vi "Create From Variant (Array).vi"(8 "error in (no error)":errorcluster, 10 "Variant":variant, 11 "JSON Value in":refnum<class "JSON Value.lvclass">) -> (0 "error out":errorcluster, 3 "JSON Value out":refnum<class "JSON Value.lvclass">)   [LabVIEW 2016, in "JSON Value.lvclass"]
doc: "Creates a new JSON instance from the given Variant."
uses:
  JSON Helper/JSON Value.lvclass
  JSON Helper/JSON Value.lvclass/JSON Value.ctl
  JSON Boolean/New JSON Boolean.vi
  JSON String/New JSON String.vi
  JSON Numeric/New JSON Numeric.vi
  <vilib>/Utility/Data Type/NI_Data Type.lvlib
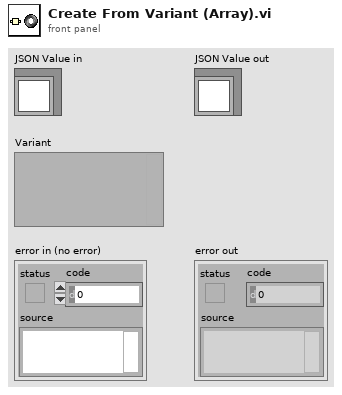
[diagram p1: front panel]
types:
  T1 = typedef "NI_Data Type.lvlib/Data Type.ctl" = enum8{"Invalid Type", "Void", "I8", "I16", "I32", "I64", "U8", "U16", "U32", "U64", "Single Float", "Double Float", "Extended Float", "Single Complex", "Double Complex", "Extended Complex", "Enum U8", "Enum U16", "Enum U32", "Enum U64", "Single Float With Unit", "Double Float With Unit", "Extended Float With Unit", "Single Complex with Unit", "Double Complex with Unit", "Extended Complex with Unit", "Boolean", "String", "Path", "Picture", "Tag", "Array", "Cluster", "Variant", "LV Variant", "Waveform", "Timestamp", "Digital Waveform", "Digital Data", "ExpressData", "Refnum", "External Data", "VI", "Poly VI", "LabVIEW Class Instance", "Fixed Point"}
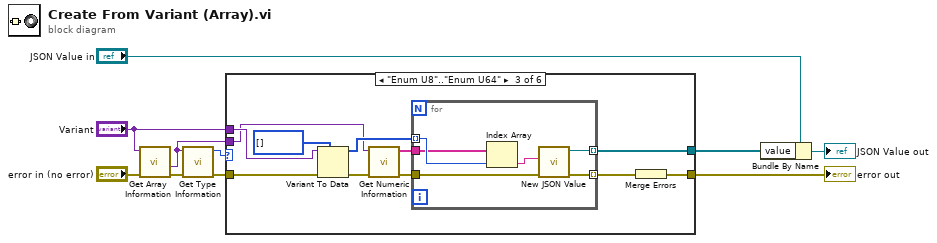
[diagram p0: block diagram]
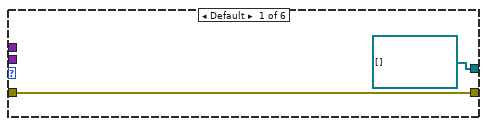
[diagram p2: hidden frame]
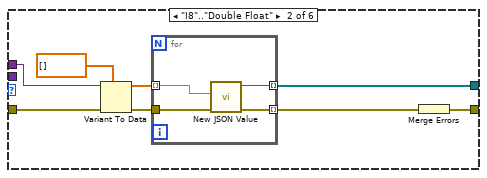
[diagram p3: hidden frame]
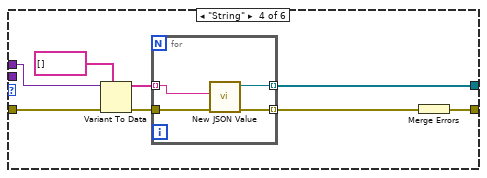
[diagram p4: hidden frame]
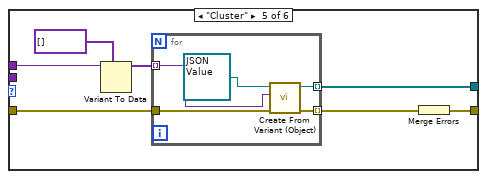
[diagram p5: hidden frame]
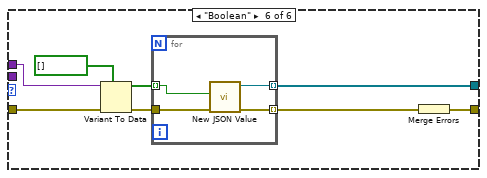
[diagram p6: hidden frame]
diagram:
  n1 = call <vilib>:"Get Array Information.vi"("error in (no error)"="error in (no error)", "Variant"="Variant") -> ("error out"=w9:errorcluster, "Array Element Data Type"=w7:variant)  [unwired: 6 in, 2 out]
  n2 = call <vilib>:"Get Type Information.vi"("error in (no error)"=w9, "Variant"=w7) -> ("error out"=w8:errorcluster, "Type"=w10:T1)  [unwired: 5 in, 3 out]
  n3 = case shown="\"Enum U8\"..\"Enum U64\"" w10 {
    tunnel: "Variant" -> [_ w19 w34 w48 w59 w72]
    tunnel: [refnum<class "JSON Value.lvclass">[] [] w13 w25 w42 w54 w66] -> w1
    tunnel: w8 -> [w12 w18 w35 w47 w56 w71]
    tunnel: [w12 w14 w26 w45 w60 w67] -> w2
    tunnel: w7 -> [_ _ w29 _ _ _]
    frame Default {
    }
    frame "I8".."Double Float" {
      n4 = Variant To Data(error in=w18, type=dbl[] [], Variant=w19) -> (data=w17:dbl[], error out=w15:errorcluster)
      n5 = for {
        tunnel: w17 -> [w24] mode=indexing
        tunnel: w15 -> [w23]
        tunnel: [w22] -> w16 mode=indexing
        tunnel: [w21] -> w13 mode=indexing
        n6 = call-poly "New JSON Value.vi"("error in (no error)"=w23, "value"=w24) -> ("error out"=w22:errorcluster, "JSON Value out"=w21:refnum<class "JSON Value.lvclass">)  [unwired: 8 in]
      }
      n7 = Merge Errors(w16) -> (w14:errorcluster)
    }
    frame "Enum U8".."Enum U64" {
      n8 = Variant To Data(error in=w35, type=u64[] [], Variant=w34) -> (data=w31:u64[], error out=w30:errorcluster)
      n9 = call <vilib>:"Get Numeric Information.vi"("error in (no error)"=w30, "Variant"=w29) -> ("error out"=w28:errorcluster, "Enum Names"=w32:string[])  [unwired: 6 in, 2 out]
      n10 = for {
        tunnel: w32 -> [w40]
        tunnel: w31 -> [w41] mode=indexing
        tunnel: w28 -> [w38]
        tunnel: [w37] -> w27 mode=indexing
        tunnel: [w36] -> w25 mode=indexing
        n11 = Index Array(array=w40, index=w41) -> (element=w39:string)
        n12 = call-poly "New JSON Value.vi"("error in (no error)"=w38, "value"=w39) -> ("error out"=w37:errorcluster, "JSON Value out"=w36:refnum<class "JSON Value.lvclass">)  [unwired: 8 in]
      }
      n13 = Merge Errors(w27) -> (w26:errorcluster)
    }
    frame "String" {
      n14 = Variant To Data(error in=w47, type=string[] [], Variant=w48) -> (data=w43:string[], error out=w46:errorcluster)
      n15 = for {
        tunnel: w43 -> [w53] mode=indexing
        tunnel: w46 -> [w52]
        tunnel: [w51] -> w44 mode=indexing
        tunnel: [w50] -> w42 mode=indexing
        n16 = call-poly "New JSON Value.vi"("error in (no error)"=w52, "value"=w53) -> ("error out"=w51:errorcluster, "JSON Value out"=w50:refnum<class "JSON Value.lvclass">)  [unwired: 8 in]
      }
      n17 = Merge Errors(w44) -> (w45:errorcluster)
    }
    frame "Cluster" {
      n18 = Variant To Data(type=variant[] [], Variant=w59) -> (data=w57:variant[])  [unwired: 1 in, 1 out]
      n19 = for {
        tunnel: w57 -> [w65] mode=indexing
        tunnel: w56 -> [w64]
        tunnel: [w63] -> w55 mode=indexing
        tunnel: [w62] -> w54 mode=indexing
        n20 = call "Create From Variant (Object).vi"("error in (no error)"=w64, "Variant"=w65, "JSON Value in"=refnum<class "JSON Value.lvclass"> refnum ("JSON Object in")) -> ("error out"=w63:errorcluster, "JSON Value out"=w62:refnum<class "JSON Value.lvclass">)  [unwired: 7 in]
      }
      n21 = Merge Errors(w55) -> (w60:errorcluster)
    }
    frame "Boolean" {
      n22 = Variant To Data(error in=w71, type=bool[] [], Variant=w72) -> (data=w70:bool[], error out=w69:errorcluster)
      n23 = for {
        tunnel: w70 -> [w77] mode=indexing
        tunnel: w69 -> [w76]
        tunnel: [w75] -> w68 mode=indexing
        tunnel: [w74] -> w66 mode=indexing
        n24 = call-poly "New JSON Value.vi"("error in (no error)"=w76, "value"=w77) -> ("error out"=w75:errorcluster, "JSON Value out"=w74:refnum<class "JSON Value.lvclass">)  [unwired: 8 in]
      }
      n25 = Merge Errors(w68) -> (w67:errorcluster)
    }
  }
  "error out" <- w2
  n26 = Bundle By Name(cluster="JSON Value in", "value"=w1) -> (→"JSON Value out":refnum<class "JSON Value.lvclass">)
